vi "Query Shutter State.vi"(8 "error in (no error)":errorcluster, 10 "Platform Slot Number (10)":i16=10 min=-1 max=255, 11 "VISA resource name":refnum<visa-resource-name>) -> (0 "error out":errorcluster, 2 "Shutter State Enabled":bool, 3 "VISA resource name out":refnum<visa-resource-name>)   [LabVIEW 2018, in "LTB-1.lvlib" / "3150.lvlib"]
doc: "Queries the state of the instrument's shutter. 0: the shutter is closed (no light is transmitted). 1: the shutter is open (allows light transmission). The shutter is used to let light through the input or block it."
uses:
  3150.lvlib
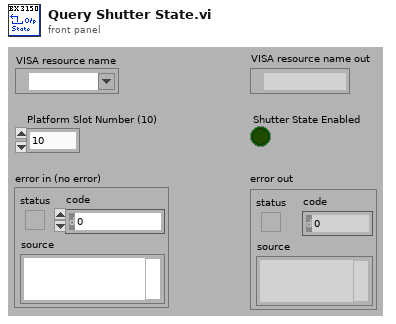
[diagram p1: front panel]
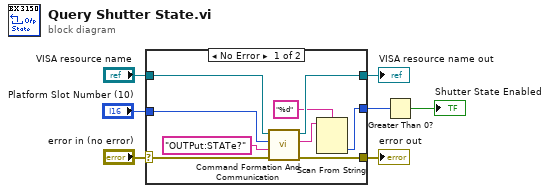
[diagram p0: block diagram]
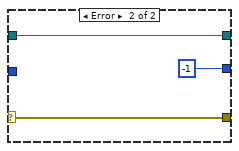
[diagram p2: hidden frame]
diagram:
  n1 = case shown="No Error" "error in (no error)" {
    selector: "error in (no error)" -> [w15 w18]
    tunnel: "VISA resource name" -> [w16 w19]
    tunnel: [w14 w19] -> w5
    tunnel: [w13 w18] -> w4
    tunnel: [w9 -1] -> w2
    tunnel: "Platform Slot Number (10)" -> [w8 _]
    frame No Error {
      n2 = call "Command Formation And Communication.vi"("error in (no error)"=w15, "Command"="OUTPut:STATe?", "Platform Slot Number"=w8, "VISA resource name"=w16) -> ("error out"=w13:errorcluster, "Response"=w10:string, "VISA resource name out"=w14:refnum<visa-resource-name>)  [unwired: 1 in, 4 out]
      n3 = Scan From String(format string="%d", input string=w10) -> (output 1=w9:i32)  [unwired: 2 in, 4 out]
    }
    frame Error {
    }
  }
  "VISA resource name out" <- w5
  "error out" <- w4
  n4 = Greater Than 0?(x=w2) -> (x > 0?=→"Shutter State Enabled":bool)
